vi "LEP_RV_ObtainRuntimeMeasurements.vi"(1 "Serial text":string) -> (0 "error out":errorcluster)   [LabVIEW 2011]
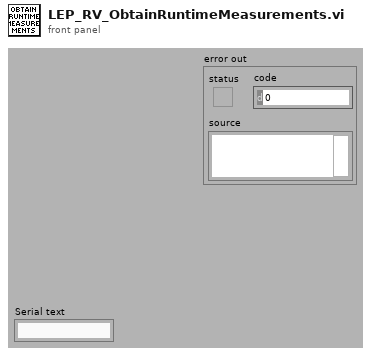
[diagram p1: front panel]
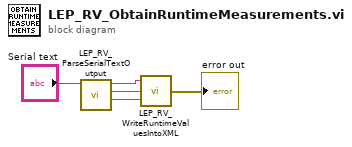
[diagram p0: block diagram]
diagram:
  n1 = call "LEP_RV_ParseSerialTextOutput.vi"("Serial text"="Serial text") -> ("Execution time"=w1:string, "Stack high water mark"=w2:string, "Heap high water mark"=w3:string)  [unwired: 4 in]
  n2 = call "LEP_RV_WriteRuntimeValuesIntoXML.vi"("Execution time"=w1, "Stack high water mark"=w2, "Heap high water mark"=w3) -> ("error out"=→"error out":errorcluster)
